vi "Stop Core.vi"(10 "final error code":i32, 11 "Cursor Digitizer in":refnum<class "Cursor Digitizer.lvclass">) -> (3 "Cursor Digitizer out":refnum<class "Cursor Digitizer.lvclass">)   [LabVIEW 2016, in "Cursor Digitizer.lvclass"]
doc: "(<B>Filename</B>: Actor Framework.lvlib:Actor.lvclass:Stop Core.vi)\n\nDefines what the actor does before it stops. Use the <B>final error code</B> input to determine whether the actor shut down in response to an error.\n\nBy default, this method does nothing. A descendant class may override it to define behavior, such as shutting down any processes the actor initiated in its override of the Actor Core method."
uses:
  Cursor Digitizer.lvclass
  Cursor Digitizer.lvclass/Cursor Digitizer.ctl
  <vilib>/ActorFramework/Actor/Actor.lvclass
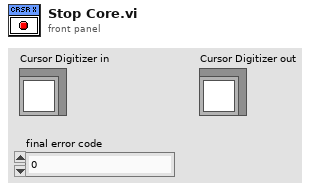
[diagram p1: front panel]
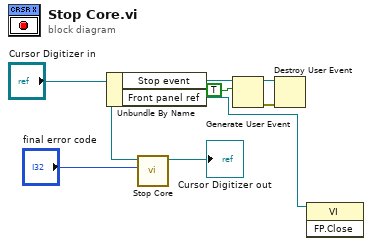
[diagram p0: block diagram]
diagram:
  n1 = Unbundle By Name("Cursor Digitizer in") -> ("Stop event"=w5:refnum<user-event>, "Front panel ref"=w1:refnum<vi>)
  n2 = call-parent "Stop Core.vi"("final error code"="final error code", "Actor in"="Cursor Digitizer in") -> ("Actor out"=→"Cursor Digitizer out":refnum<class "Cursor Digitizer.lvclass">)  [unwired: 9 in]
  n3 = Generate User Event(user event=w5, event data cluster=TRUE ("event data")) -> (user event out=w2:refnum<user-event>, error out=w3:errorcluster)  [unwired: 2 in]
  n4 = Destroy User Event(user event=w2, error in=w3) -> ()  [unwired: 1 out]
  n5 = invoke class="VI" method="FP.Close"(reference=w1) -> ()  [unwired: 2 in, 3 out]
